vi "PH_ImageOperator.TraceAnalysis.vi"(0 "i ref in":refnum<vi>, 5 "error in (no error)":errorcluster) -> (14 "i ref out":refnum<vi>, 19 "error out":errorcluster)   [LabVIEW 2014, in "PH_ImageOperator.lvlib"]
doc: "This VI does several calculations related to the major and minor beam trace."
uses:
  PH_ImageOperator.lvlib
  PH_StatusHandler/PH_StatusHandler.Status.ctl
  PH_StatusHandler/PH_StatusHandler.lvlib
panel:
  in  "Trace":T1
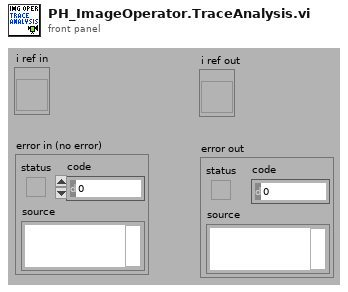
[diagram p1: front panel]
types:
  T1 = cluster{"XScaleName":string, "Y Scale Minimum":sgl, "Y Scale Maximum":sgl, "X Scale Minimum":sgl, "X Scale Maximum":sgl, "Traces":cluster{"Index":sgl[], "Trace":dbl[]}[]}
  T2 = typedef "PH_StatusHandler.lvlib/PH_StatusHandler.Status.ctl" = i16
  T3 = typedef "PH_ImageOperator.lvlib/PH_ImageOperator.i attribute.ctl" = cluster{"GUI Refs":cluster{"Delete":refnum<vi>, "Calibration status":refnum<vi>, "BI subtracted":refnum<vi>, "calc Energy":refnum<vi>, "Energy: expected value":refnum<vi>, "Energy: Tolerance":refnum<vi>, "Energy calculated":refnum<vi>, "Energy":refnum<vi>, "calc Beam Anal":refnum<vi>, "Maj Diam 1/esquare":refnum<vi>, "Min Diam 1/esquare":refnum<vi>, "Azi Angle":refnum<vi>, "Min/Maj Diam esquare":refnum<vi>, "Beam analysed":refnum<vi>, "CoG - x":refnum<vi>, "CoG - y":refnum<vi>, "BA: Method":refnum<vi>, "BA: Steps":refnum<vi>, "BA: Factor":refnum<vi>, "calc Traces":refnum<vi>, "Traces: Fit Gauss":refnum<vi>, "Traces calculated":refnum<vi>, "Maj FWHM":refnum<vi>, "Min FWHM":refnum<vi>, "Major Trace":refnum<vi>, "Minor Trace":refnum<vi>, "Maj Fit Order":refnum<vi>, "Min Fit Order":refnum<vi>, "Position calculated":refnum<vi>, "Position":refnum<vi>, "Type":refnum<vi>, "Center":refnum<vi>, "exp - X":refnum<vi>, "exp - Y":refnum<vi>, "Tolerance":refnum<vi>, "f":refnum<vi>, "M":refnum<vi>, "D":refnum<vi>, "q":refnum<vi>, "Dummy Method":refnum<vi>, "Dummy Type":refnum<vi>, "Global On":refnum<vi>, "Traces: No offset":refnum<vi>, "Maj 99%":refnum<vi>, "Min 99%":refnum<vi>, "GUI FF Image":refnum<vi>, "calc Fill Factor":refnum<vi>, "FF calculated":refnum<vi>, "Fill Factor: Filter?":refnum<vi>, "FF: Damage Threshold":refnum<vi>, "FF: Threshold":refnum<vi>, "FF: max allow. Energy":refnum<vi>, "FF: Fillfactor":refnum<vi>, "Calibration data":refnum<vi>}, "List of GUIs":string[], "Calibration":cluster{"Status":T2, "Calibration data":T4, "Calibration Data File":path}, "Final Image":cluster{"BI Subtraction Failure":bool}, "Energy":cluster{"on":bool, "expected value [mJ]":dbl, "Tolerance [%]":dbl, "State":T2, "Energy [mJ]":dbl, "Unit":string, "calculated @":timestamp}, "Beam Analysis":cluster{"on":bool, "Data":T5, "Method":bool, "Steps":i32, "Factor":i32, "ROI":cluster{"Left":i32, "Top":i32, "Right":i32, "Bottom":i32}, "analysed @":timestamp}, "Trace Analysis":cluster{"on":bool, "Fit on":bool, "Maj FWHM":dbl, "Min FWHM":dbl, "Maj Fit Order":i32, "Min Fit Order":i32, "No Offset":bool, "Maj 99%":dbl, "Min 99%":dbl, "Traces":cluster{"XScaleName":string, "Y Scale Minimum":sgl, "Y Scale Maximum":sgl, "X Scale Minimum":sgl, "X Scale Maximum":sgl, "Traces":cluster{"Index":sgl[], "Trace":dbl[]}[]}[], "analysed @":timestamp}, "Position Analysis":cluster{"on":bool, "exp - X":i32, "exp - Y":i32, "focal length [mm]":dbl, "Magnification":dbl, "Delta":dbl, "Theta":dbl, "Tolerance":dbl, "Type":bool, "analysed @":timestamp}, "Fill Factor":cluster{"on":bool, "Filter on?":bool, "Threshold":dbl, "Damage Threshold [J/cm²]":dbl, "Fillfactor":dbl, "Max. allowed Energy [J]":dbl, "calculated @":timestamp}, "Statistician Service ID":i32, "Images":cluster{"Background":T6, "OP":T6, "GUI":T6, "BA: ROI":T6, "Trace: Turn":T6, "FF: Main":T6, "FF: Help":T6, "PSDB: BG":T6, "PSDB: OP":T6, "PSDB: FF":T6}}
  T4 = typedef "PH_ImageCalibrator.lvlib/PH_ImageCalibrator.Calibration Data.ctl" = cluster{"Date":string, "Time":string, "Cam Settings":cluster{"Cam ID":string, "Gain":dbl, "Brightness":dbl, "Shutter":dbl, "Cam Error":bool, "Mode":i32}, "Background Image":cluster{"Image":dbl[][], "Image Error":bool}, "Linear Calibration":cluster{"Calibration Factor":dbl, "not mm or mrad":bool}, "Energy Calibration":cluster{"Calibration Factor":dbl, "no mJ":bool}}
  T5 = typedef "PH_ImageOperator.lvlib/PH_ImageOperator.Beam Analysis Data.ctl" = cluster{"CoG-x":sgl, "CoG-y":sgl, "Maj Dim":dbl, "Min Dim":dbl, "Ellipticity":dbl, "Azimuth Angle [rad]":dbl, "Azi Angle rel to Maj?":bool}
  T6 = typedef "IMAQ Image.ctl" = refnum<image>
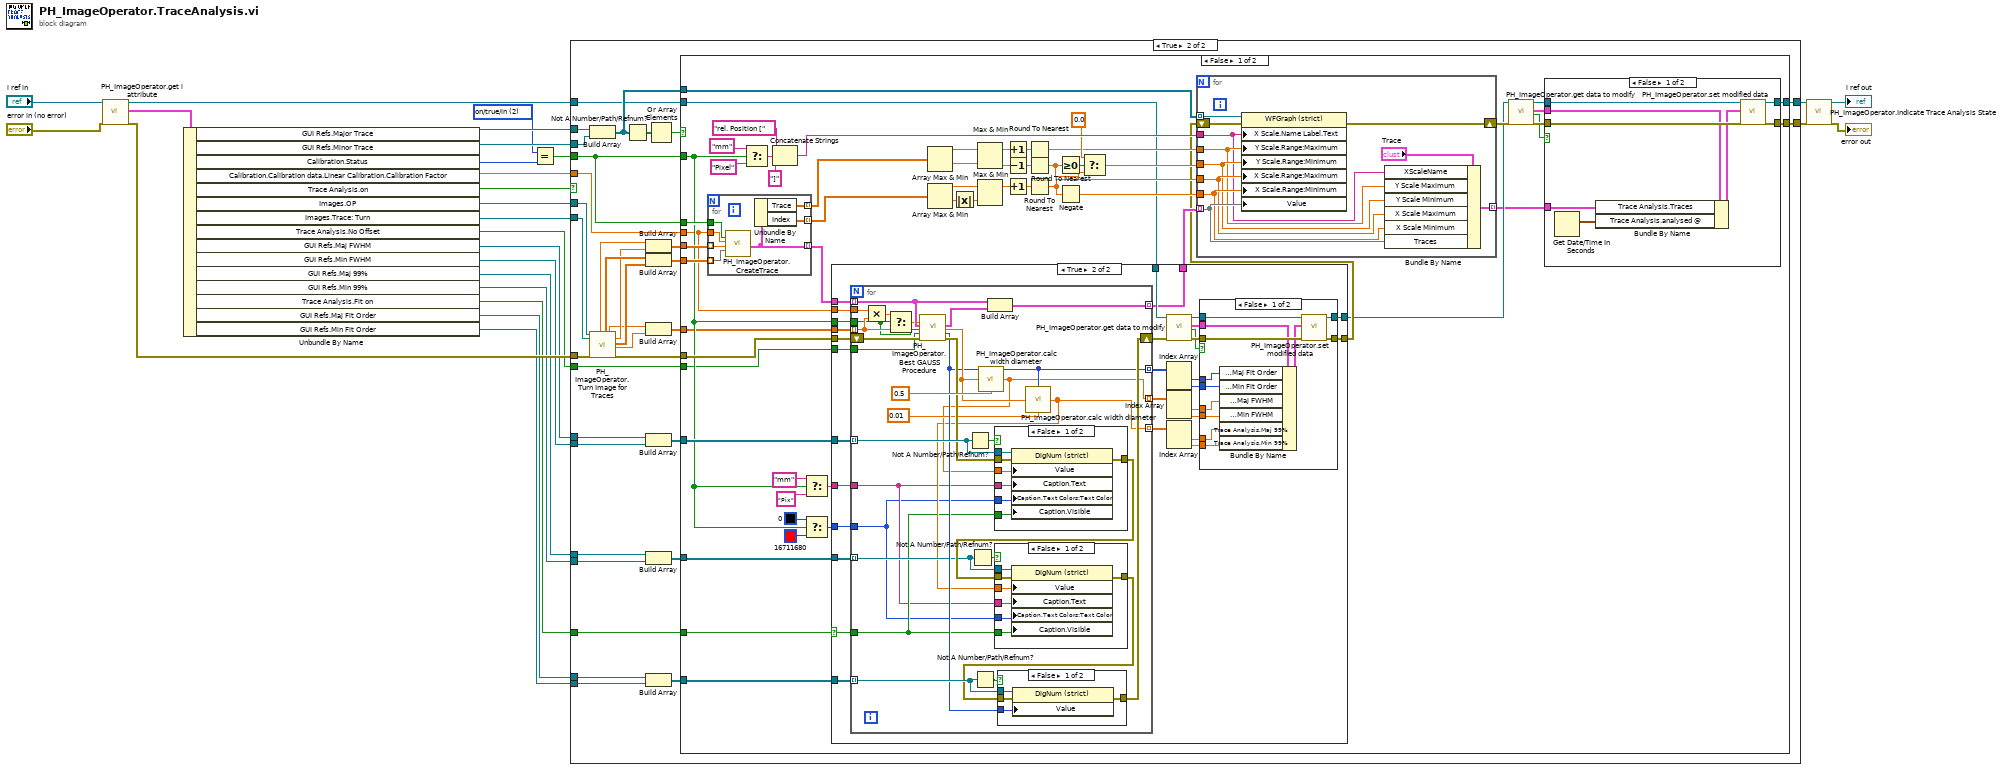
[diagram p0: block diagram]
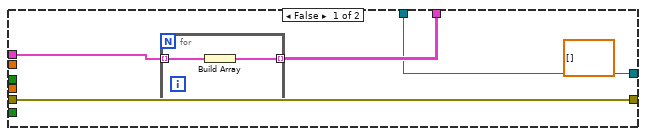
[diagram p4: hidden frame]
diagram:
  w16 = T2 2 items=["no info", "off/false/out", "on/true/in", "Failure", "Alarm", "Status 1", "Status 2", "Status 3"] ("Calibration.Status")
  n1 = call "PH_ImageOperator.get i attribute.vi"("i ref in"="i ref in", "error in (no error)"="error in (no error)") -> ("i ref out"=w23:refnum<vi>, "i attribute"=w26:T3, "error out"=w21:errorcluster)  [unwired: 15 in]
  n2 = Unbundle By Name(w26) -> ("GUI Refs.Major Trace"=w20:refnum<vi>, "GUI Refs.Minor Trace"=w19:refnum<vi>, "Calibration.Status"=w17:T2, "Calibration.Calibration data.Linear Calibration.Calibration Factor"=w18:dbl, "Trace Analysis.on"=w22:bool, "Images.OP"=w2:T6, "Images.Trace: Turn"=w1:T6, "Trace Analysis.No Offset"=w6:bool, "GUI Refs.Maj FWHM"=w7:refnum<vi>, "GUI Refs.Min FWHM"=w14:refnum<vi>, "GUI Refs.Maj 99%"=w4:refnum<vi>, "GUI Refs.Min 99%"=w3:refnum<vi>, "Trace Analysis.Fit on"=w5:bool, "GUI Refs.Maj Fit Order"=w13:refnum<vi>, "GUI Refs.Min Fit Order"=w12:refnum<vi>)
  n3 = Equal?(x=w16, y=w17) -> (x = y?=w15:bool)
  n4 = case shown="True" w22 {
    tunnel: [w27 w56] -> w9
    tunnel: w2 -> [_ w46]
    tunnel: w1 -> [_ w47]
    tunnel: w23 -> [w28 w34]
    tunnel: [w28 w33] -> w10
    tunnel: w21 -> [w27 w62]
    tunnel: w20 -> [_ w61]
    tunnel: w19 -> [_ w60]
    tunnel: w18 -> [_ w49]
    tunnel: w15 -> [_ w48]
    tunnel: w7 -> [_ w41]
    tunnel: w14 -> [_ w40]
    tunnel: w13 -> [_ w39]
    tunnel: w12 -> [_ w38]
    tunnel: w5 -> [_ w35]
    tunnel: w6 -> [_ w32]
    tunnel: w4 -> [_ w30]
    tunnel: w3 -> [_ w29]
    frame False {
    }
    frame True {
      n5 = Build Array(w61, w60) -> (w57:refnum<vi>[])
      n6 = call "PH_ImageOperator.Turn Image for Traces.vi"("Operation Image"=w46, "Turn Image in"=w47, "error in (no error)"=w62) -> ("Major Offset"=w53:sgl, "Major Trace"=w54:sgl[], "Maj Dim"=w44:dbl, "Minor Offset"=w52:sgl, "Minor Trace"=w55:sgl[], "Min Dim"=w43:dbl, "error out"=w45:errorcluster)  [unwired: 10 in]
      n7 = Not A Number/Path/Refnum?(number/path/refnum=w57) -> (NaN/Path/Refnum?=w59:bool[])
      n8 = Build Array(w53, w52) -> (w50:sgl[])
      n9 = Build Array(w54, w55) -> (w51:sgl[][])
      n10 = Build Array(w44, w43) -> (w42:dbl[])
      n11 = Build Array(w41, w40) -> (w36:refnum<vi>[])
      n12 = Build Array(w30, w29) -> (w31:refnum<vi>[])
      n13 = Build Array(w39, w38) -> (w37:refnum<vi>[])
      n14 = Or Array Elements(Boolean array=w59) -> (logical OR=w58:bool)
      n15 = case shown="False" w58 {
        tunnel: w57 -> [w120 _]
        tunnel: [w69 w250] -> w56
        tunnel: w51 -> [w119 _]
        tunnel: w50 -> [w118 _]
        tunnel: w48 -> [w117 _]
        tunnel: w49 -> [w75 _]
        tunnel: w48 -> [w76 _]
        tunnel: w45 -> [w90 w250]
        tunnel: w42 -> [w72 _]
        tunnel: w37 -> [w87 _]
        tunnel: w36 -> [w86 _]
        tunnel: w35 -> [w83 _]
        tunnel: w34 -> [w82 w249]
        tunnel: [w66 w249] -> w33
        tunnel: w32 -> [w74 _]
        tunnel: w31 -> [w73 _]
        frame False {
          n16 = for {
            tunnel: w119 -> [w237] mode=indexing
            tunnel: w118 -> [w236] mode=indexing
            tunnel: w117 -> [w235]
            tunnel: w75 -> [w234]
            tunnel: [w233] -> w89 mode=indexing
            tunnel: [w232] -> w94 mode=indexing
            tunnel: [w231] -> w103 mode=indexing
            n17 = call "PH_ImageOperator.CreateTrace.vi"("Calibrate"=w235, "Calibration Factor"=w234, "Offset"=w236, "Trace"=w237) -> ("Trace Output"=w233:cluster{"Index":sgl[], "Trace":sgl[]})  [unwired: 14 in, 1 out]
            n18 = Unbundle By Name(w233) -> ("Trace"=w231:sgl[], "Index"=w232:sgl[])
          }
          n19 = Select(t="mm", s=w76, f="Pixel" ("string")) -> (s? t:f=w115:string)
          n20 = Concatenate Strings("rel. Position [" ("string"), w115, "]" ("string")) -> (w111:string)
          n21 = Select(t="mm", s=w76, f="Pix" ("string")) -> (s? t:f=w81:string)
          n22 = Select(t=u32 0 ("Color"), s=w76, f=u32 16711680 ("Color")) -> (s? t:f=w80:u32)
          n23 = case shown="True" w83 {
            selector: w83 -> [_ w145]
            tunnel: w90 -> [w132 w166]
            tunnel: [w132 w155] -> w77
            tunnel: w72 -> [_ w165]
            tunnel: w89 -> [w134 w164]
            tunnel: [w133 w137] -> w88
            tunnel: w87 -> [_ w163]
            tunnel: w86 -> [_ w162]
            tunnel: w81 -> [_ w161]
            tunnel: w82 -> [w131 w149]
            tunnel: [w131 w148] -> w67
            tunnel: w80 -> [_ w146]
            tunnel: w76 -> [_ w144]
            tunnel: w75 -> [_ w143]
            tunnel: w74 -> [_ w142]
            tunnel: w73 -> [_ w138]
            frame False {
              (unwired) dbl[][] [] ("mse array")
              n24 = for {
                tunnel: w134 -> [w136] mode=indexing
                tunnel: [w135] -> w133 mode=indexing
                n25 = Build Array(w136) -> (w135:cluster{"Index":sgl[], "Trace":sgl[]}[])
              }
            }
            frame True {
              n26 = for {
                shift-right: [w197] -> w156
                shift-left: w166 -> [w209]
                tunnel: w165 -> [w201] mode=indexing
                tunnel: w164 -> [w204] mode=indexing
                tunnel: w163 -> [w195] mode=indexing
                tunnel: w162 -> [w196] mode=indexing
                tunnel: w161 -> [w182]
                tunnel: [w205] -> w137 mode=indexing
                tunnel: [w189] -> w154 mode=indexing
                tunnel: [w191] -> w150 mode=indexing
                tunnel: w146 -> [w181]
                tunnel: w145 -> [w183]
                tunnel: w144 -> [w199]
                tunnel: w143 -> [w200]
                tunnel: w142 -> [w198]
                tunnel: [w184] -> w140 mode=indexing
                tunnel: w138 -> [w185] mode=indexing
                n27 = Multiply(x=w200, y=w201) -> (x*y=w202:dbl)
                n28 = Select(t=w202, s=w199, f=w201) -> (s? t:f=w203:dbl)
                n29 = call "PH_ImageOperator.Best GAUSS Procedure.vi"("Diameter"=w203, "Data Trace"=w204, "calibrated?"=w199, "No Offset?"=w198, "error in (no error)"=w209) -> ("Best Fit Trace"=w206:cluster{"Index":sgl[], "Best Fit":dbl[]}, "Best Fit Width Parameter"=w192:dbl, "Best Fit Order"=w191:i32, "error out"=w193:errorcluster)  [unwired: 11 in]
                n30 = Not A Number/Path/Refnum?(number/path/refnum=w196) -> (NaN/Path/Refnum?=w207:bool)
                n31 = Not A Number/Path/Refnum?(number/path/refnum=w185) -> (NaN/Path/Refnum?=w188:bool)
                n32 = Not A Number/Path/Refnum?(number/path/refnum=w195) -> (NaN/Path/Refnum?=w208:bool)
                n33 = call "PH_ImageOperator.calc width diameter.vi"("Best Fit Order"=w191, "Percent"=0.5, "Best Fit Width Parameter"=w192) -> ("Result"=w189:dbl)  [unwired: 12 in]
                n34 = Build Array(w204, w206) -> (w205:cluster{"Index":sgl[], "Best Fit":dbl[]}[])
                n35 = case shown="False" w207 {
                  tunnel: w196 -> [w229 _]
                  tunnel: w189 -> [w228 _]
                  tunnel: w193 -> [w227 w230]
                  tunnel: [w226 w230] -> w187
                  tunnel: w182 -> [w225 _]
                  tunnel: w181 -> [w224 _]
                  tunnel: w183 -> [w223 _]
                  frame False {
                    n36 = property class="DigNum (strict)"(reference=w229, error in=w227, "Value"=w228, "Caption.Text"=w225, "Caption.Text Colors:Text Color"=w224, "Caption.Visible"=w223) -> (error out=w226:errorcluster)  [unwired: 1 out]
                  }
                  frame True {
                  }
                }
                n37 = call "PH_ImageOperator.calc width diameter.vi"("Best Fit Order"=w191, "Percent"=0.01, "Best Fit Width Parameter"=w192) -> ("Result"=w184:dbl)  [unwired: 12 in]
                n38 = case shown="False" w188 {
                  tunnel: w185 -> [w216 _]
                  tunnel: w184 -> [w215 _]
                  tunnel: w187 -> [w214 w217]
                  tunnel: [w213 w217] -> w186
                  tunnel: w182 -> [w212 _]
                  tunnel: w181 -> [w211 _]
                  tunnel: w183 -> [w210 _]
                  frame False {
                    n39 = property class="DigNum (strict)"(reference=w216, error in=w214, "Value"=w215, "Caption.Text"=w212, "Caption.Text Colors:Text Color"=w211, "Caption.Visible"=w210) -> (error out=w213:errorcluster)  [unwired: 1 out]
                  }
                  frame True {
                  }
                }
                n40 = case shown="False" w208 {
                  tunnel: w195 -> [w221 _]
                  tunnel: w191 -> [w220 _]
                  tunnel: [w219 w222] -> w197
                  tunnel: w186 -> [w218 w222]
                  frame False {
                    n41 = property class="DigNum (strict)"(reference=w221, error in=w218, "Value"=w220) -> (error out=w219:errorcluster)  [unwired: 1 out]
                  }
                  frame True {
                  }
                }
              }
              n42 = call "PH_ImageOperator.get data to modify.vi"("i ref in"=w149, "error in (no error)"=w156) -> ("i ref out"=w160:refnum<vi>, "i attribute"=w158:T3, "timed out"=w157:bool, "error out"=w159:errorcluster)  [unwired: 14 in]
              n43 = Index Array(array=w150) -> (element #1=w151:i32, element #2=w147:i32)  [unwired: 2 in]
              n44 = Index Array(array=w154) -> (element #1=w153:dbl, element #2=w152:dbl)  [unwired: 2 in]
              n45 = Index Array(array=w140) -> (element #1=w141:dbl, element #2=w139:dbl)  [unwired: 2 in]
              n46 = case shown="False" w157 {
                tunnel: w160 -> [w178 w180]
                tunnel: [w177 w180] -> w148
                tunnel: w159 -> [w176 w179]
                tunnel: [w175 w179] -> w155
                tunnel: w158 -> [w174 _]
                tunnel: w153 -> [w169 _]
                tunnel: w152 -> [w170 _]
                tunnel: w151 -> [w172 _]
                tunnel: w147 -> [w171 _]
                tunnel: w141 -> [w168 _]
                tunnel: w139 -> [w167 _]
                frame False {
                  n47 = Bundle By Name(cluster=w174, "Trace Analysis.Maj Fit Order"=w172, "Trace Analysis.Min Fit Order"=w171, "Trace Analysis.Maj FWHM"=w169, "Trace Analysis.Min FWHM"=w170, "Trace Analysis.Maj 99%"=w168, "Trace Analysis.Min 99%"=w167) -> (w173:T3)
                  n48 = call "PH_ImageOperator.set modified data.vi"("i ref in"=w178, "i attribute"=w173, "error in (no error)"=w176) -> ("i ref out"=w177:refnum<vi>, "error out"=w175:errorcluster)  [unwired: 15 in]
                }
                frame True {
                }
              }
            }
          }
          n49 = Array Max & Min(array=w103) -> (max value=w110:sgl, min value=w100:sgl)  [unwired: 2 out]
          n50 = Array Max & Min(array=w94) -> (max value=w97:sgl, min value=w99:sgl)  [unwired: 2 out]
          n51 = Absolute Value(x=w99) -> (abs(x)=w98:sgl)
          n52 = Max & Min(x=w110, y=w100) -> (max(x,y)=w109:sgl, min(x,y)=w106:sgl)
          n53 = Max & Min(x=w97, y=w98) -> (max(x,y)=w96:sgl)  [unwired: 1 out]
          n54 = Increment(x=w109) -> (x+1=w108:sgl)
          n55 = Decrement(x=w106) -> (x-1=w107:sgl)
          n56 = Increment(x=w96) -> (x+1=w95:sgl)
          n57 = Round To Nearest(number=w108) -> (nearest integer value=w102:sgl)
          n58 = Round To Nearest(number=w107) -> (nearest integer value=w91:sgl)
          n59 = Round To Nearest(number=w95) -> (nearest integer value=w93:sgl)
          n60 = Greater Or Equal To 0?(x=w91) -> (x >= 0?=w105:bool)
          n61 = Negate(x=w93) -> (-x=w92:sgl)
          n62 = Select(t=0.0, s=w105, f=w91) -> (s? t:f=w101:dbl)
          n63 = for {
            tunnel: w120 -> [w247] mode=indexing
            shift-right: [w246] -> w70
            shift-left: w77 -> [w248]
            tunnel: w88 -> [w244] mode=indexing
            tunnel: w111 -> [w239]
            tunnel: w102 -> [w240]
            tunnel: w101 -> [w241]
            tunnel: w93 -> [w242]
            tunnel: w92 -> [w243]
            tunnel: [w238] -> w63 mode=indexing
            n64 = property on="Property Node" class="WFGraph (strict)"(reference=w247, error in=w248, "X Scale.Name Label.Text"=w239, "Y Scale.Range:Maximum"=w240, "Y Scale.Range:Minimum"=w241, "X Scale.Range:Maximum"=w242, "X Scale.Range:Minimum"=w243, "Value"=w244) -> (error out=w246:errorcluster)  [unwired: 1 out]
            n65 = Bundle By Name(cluster="Trace", "XScaleName"=w239, "Y Scale Maximum"=w240, "Y Scale Minimum"=w241, "X Scale Maximum"=w242, "X Scale Minimum"=w243, "Traces"=w244) -> (w238:T1)
          }
          n66 = call "PH_ImageOperator.get data to modify.vi"("i ref in"=w67, "error in (no error)"=w70) -> ("i ref out"=w68:refnum<vi>, "i attribute"=w64:T3, "timed out"=w65:bool, "error out"=w71:errorcluster)  [unwired: 14 in]
          n67 = case shown="False" w65 {
            tunnel: w71 -> [w128 w129]
            tunnel: [w127 w129] -> w69
            tunnel: w68 -> [w126 w130]
            tunnel: [w125 w130] -> w66
            tunnel: w64 -> [w124 _]
            tunnel: w63 -> [w122 _]
            frame False {
              n68 = Get Date/Time In Seconds() -> (seconds since 1Jan1904=w121:timestamp)
              n69 = Bundle By Name(cluster=w124, "Trace Analysis.Traces"=w122, "Trace Analysis.analysed @"=w121) -> (w123:T3)
              n70 = call "PH_ImageOperator.set modified data.vi"("i ref in"=w126, "i attribute"=w123, "error in (no error)"=w128) -> ("i ref out"=w125:refnum<vi>, "error out"=w127:errorcluster)  [unwired: 15 in]
            }
            frame True {
            }
          }
        }
        frame True {
        }
      }
    }
  }
  n71 = call "PH_ImageOperator.Indicate Trace Analysis State.vi"("i ref in"=w10, "error in (no error)"=w9) -> ("i ref out"=→"i ref out":refnum<vi>, "error out"=→"error out":errorcluster)  [unwired: 16 in]
